vi "process.vi"(11 "class":refnum<class "selection_dropdown.lvclass">) -> ()   [LabVIEW 2024, in "selection_dropdown.lvclass"]
uses:
  selection_dropdown.lvclass
  refs.ctl
  selection_dropdown.lvclass/selection_dropdown.ctl
  <vilib>/addons/_JKI Toolkits/State Machine/_JKI_lib_State_Machine.llb/Select State(s)_err__jki_lib_state_machine.vi
  6cc69b80-9b04-4322-8415-f8fc40951971.vi
  <vilib>/addons/_JKI Toolkits/State Machine/_JKI_lib_State_Machine.llb/Periodic Trigger__ogtk__JKI-SM__jki_lib_state_machine.vi
  <vilib>/ErrorRing/Error Ring.xnode
panel:
  in  "Exit":bool
  in  "error in (no error)":errorcluster
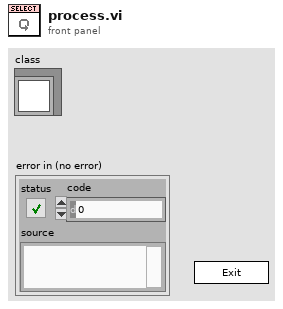
[diagram p1: front panel]
types:
  T1 = enum32{"Invalid", "Standard", "Closed", "Hidden", "Minimized", "Maximized"}
  T2 = enum32{"invalid app kind", "Development System", "Run Time System", "Student Edition", "Embedded LabVIEW", "Evaluation", "Custom"}
  T3 = typedef "selection_dropdown.lvclass/refs.ctl" = cluster{"selection":refnum<vi>, "cancel":refnum<vi>, "list":refnum<vi>, "available":refnum<vi>, "delete":refnum<vi>, "delete all":refnum<vi>}
  T4 = cluster{"Core":cluster{"Current VI Reference":refnum<vi>, "Close Panel on Exit?":bool}, "class":refnum<class "selection_dropdown.lvclass">, "refs":T3, "avail set":string[]}
  T5 = cluster{"Current VI Reference":refnum<vi>, "Close Panel on Exit?":bool}
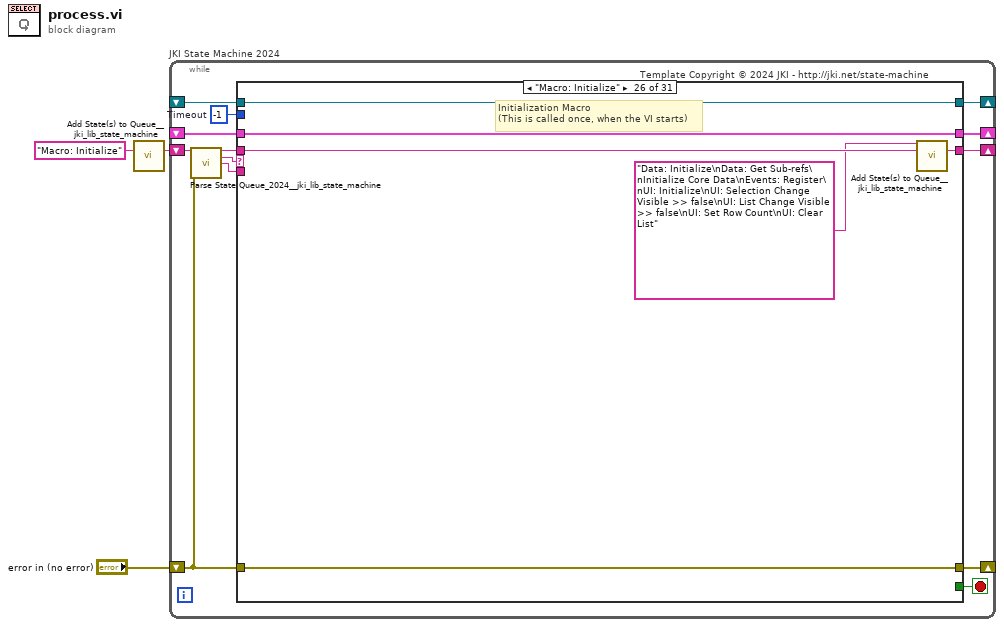
[diagram p0: block diagram]
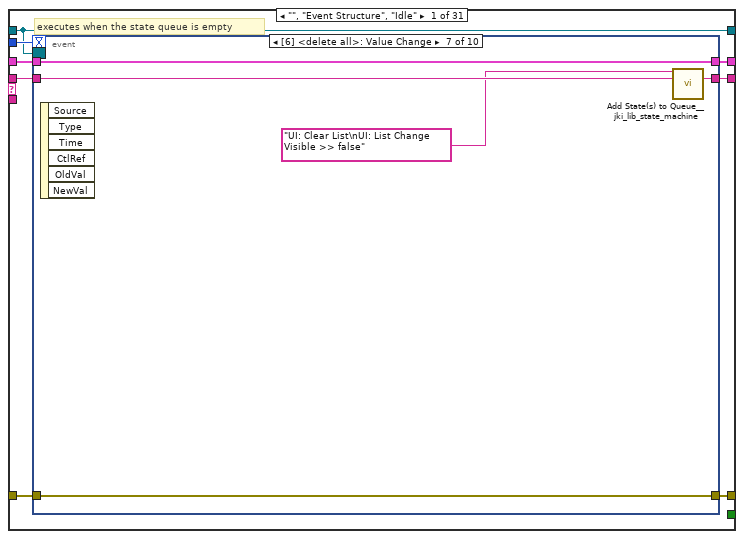
[diagram p2: hidden frame]
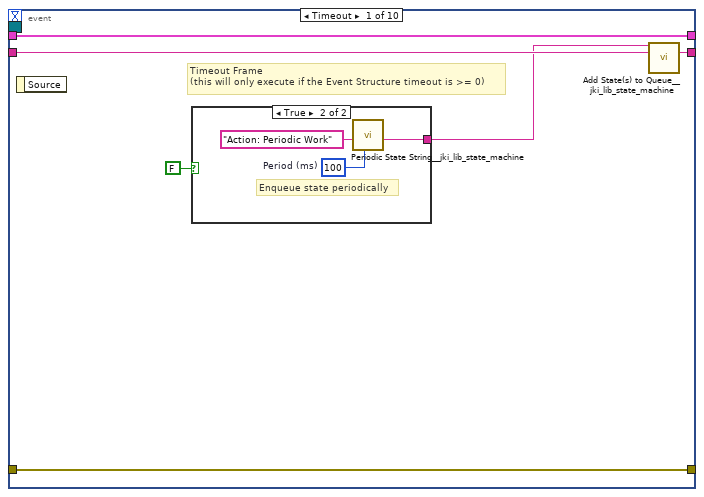
[diagram p3: hidden frame]
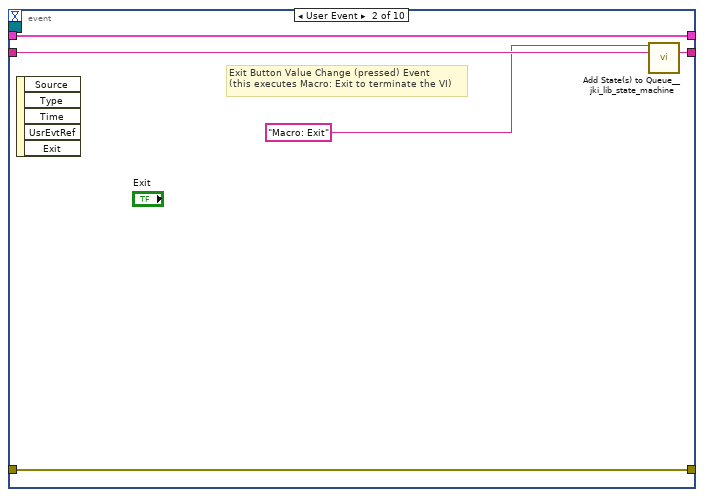
[diagram p5: hidden frame]
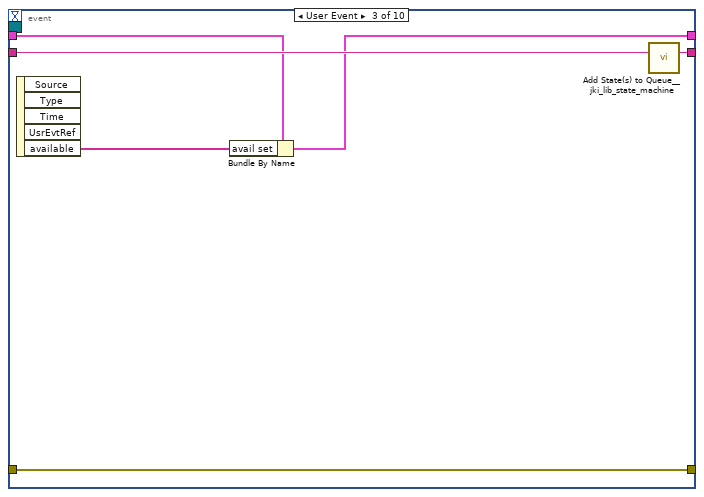
[diagram p6: hidden frame]
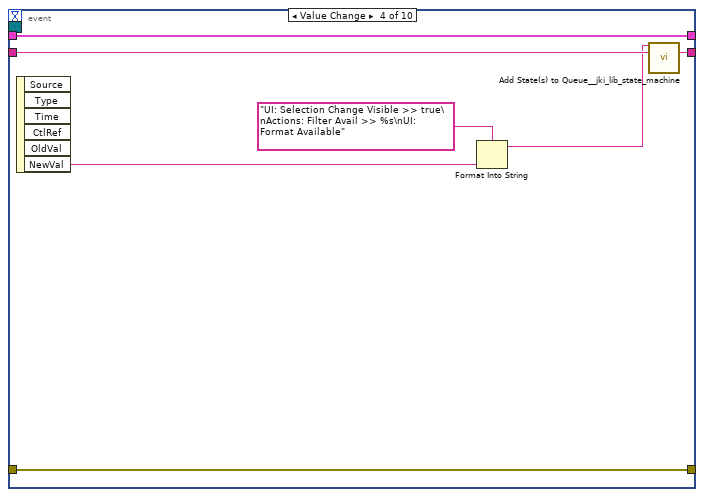
[diagram p7: hidden frame]
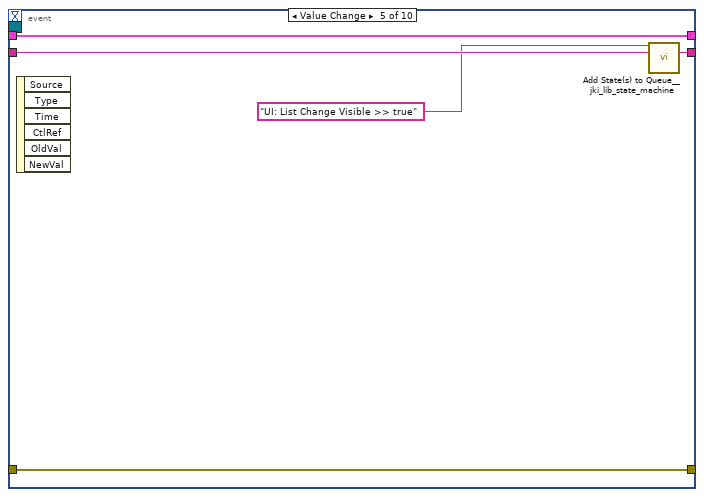
[diagram p8: hidden frame]
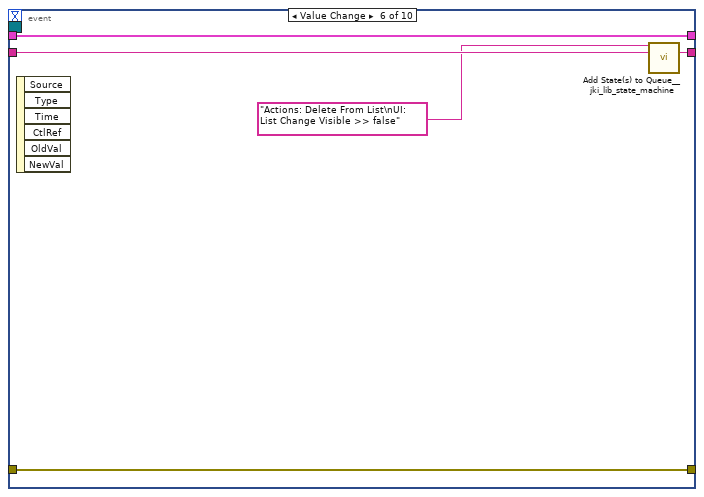
[diagram p9: hidden frame]
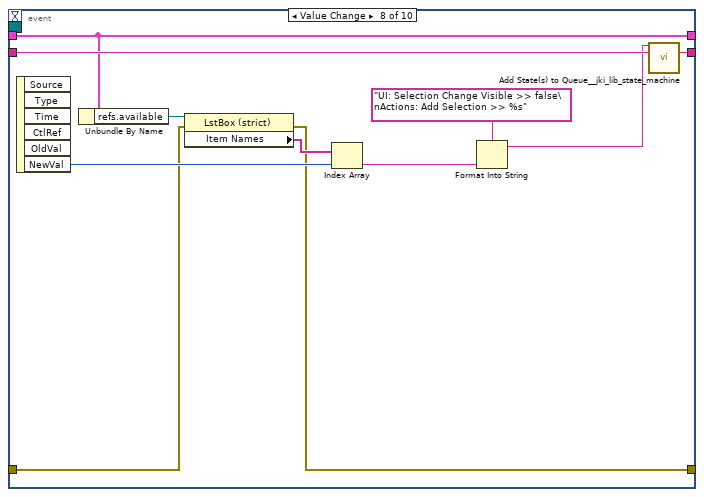
[diagram p10: hidden frame]
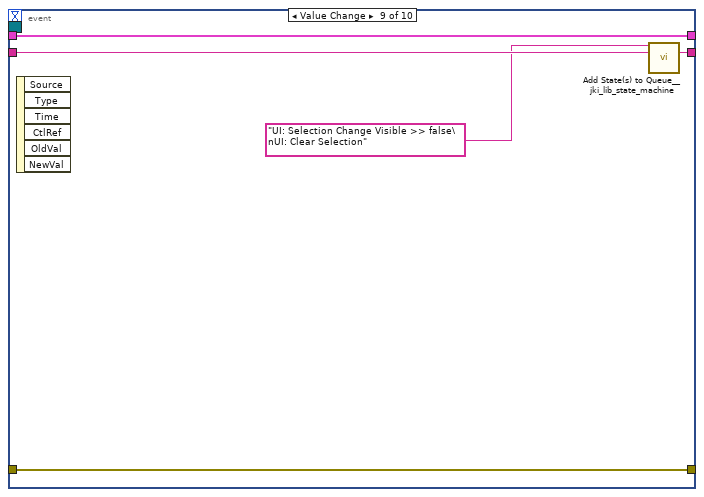
[diagram p11: hidden frame]
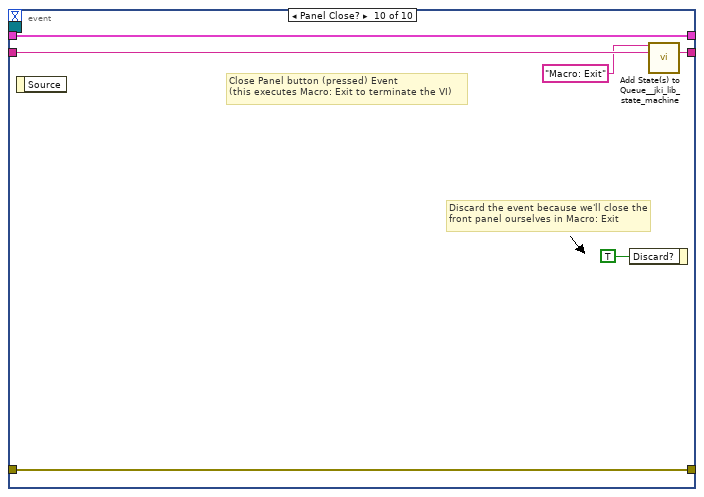
[diagram p12: hidden frame]
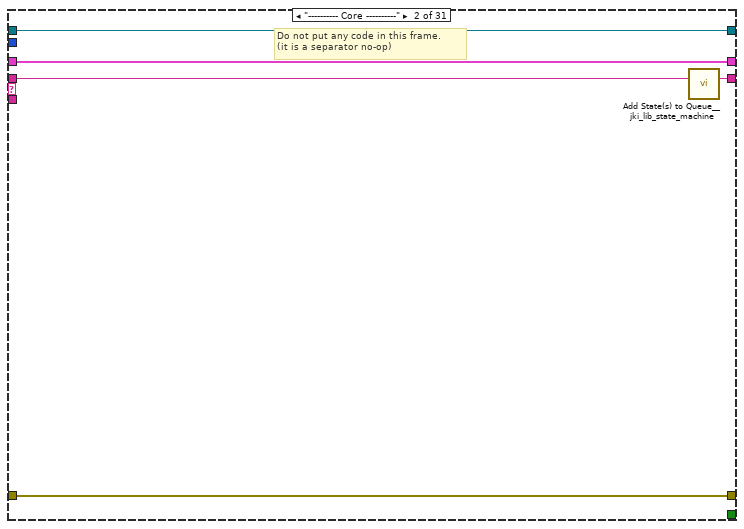
[diagram p13: hidden frame]
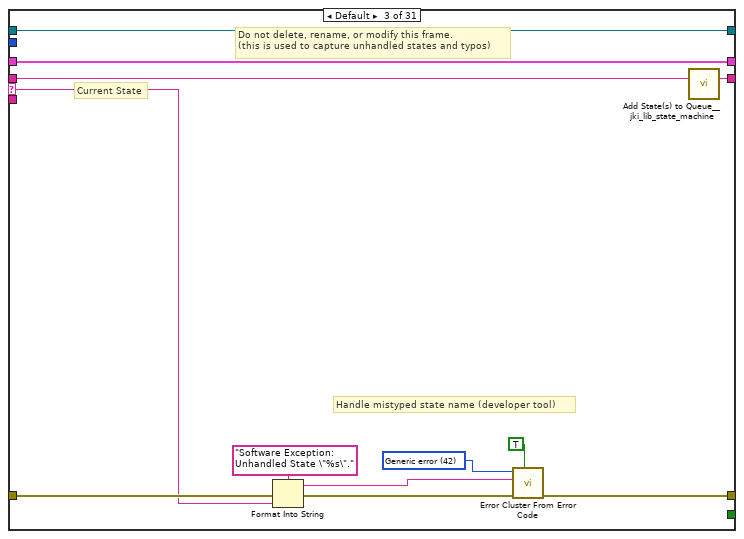
[diagram p14: hidden frame]
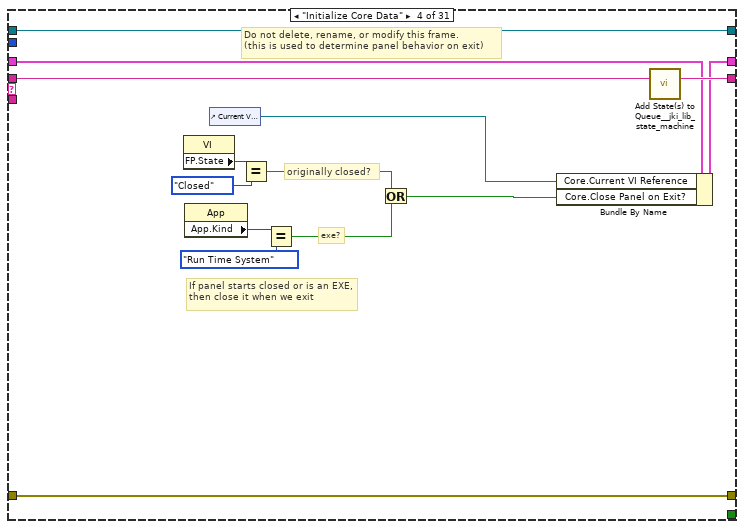
[diagram p15: hidden frame]
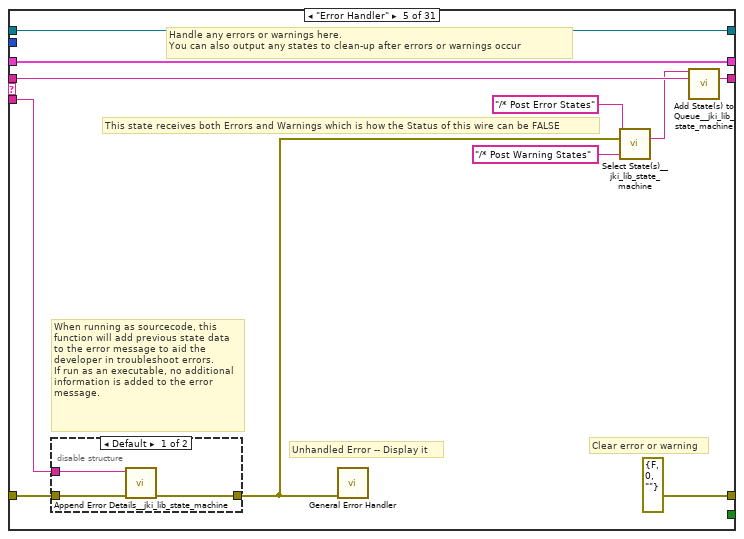
[diagram p16: hidden frame]
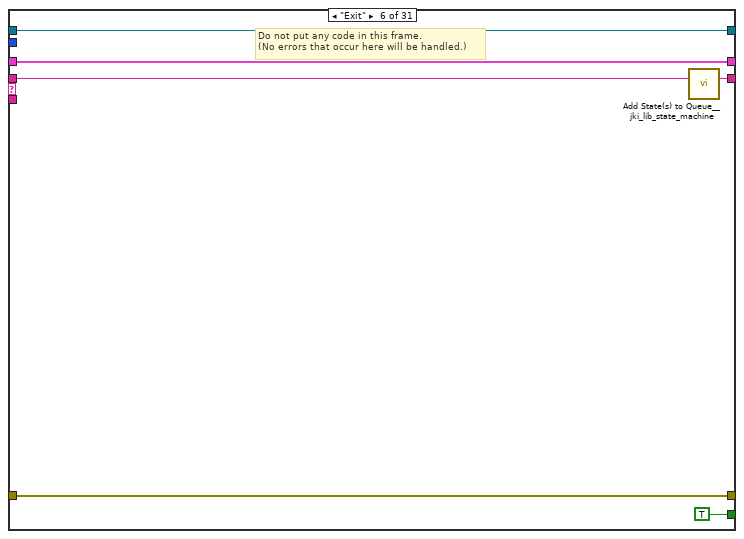
[diagram p18: hidden frame]
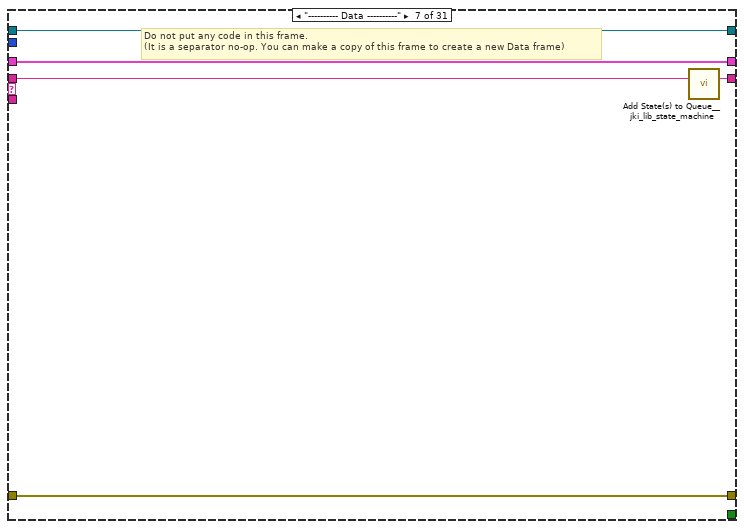
[diagram p19: hidden frame]
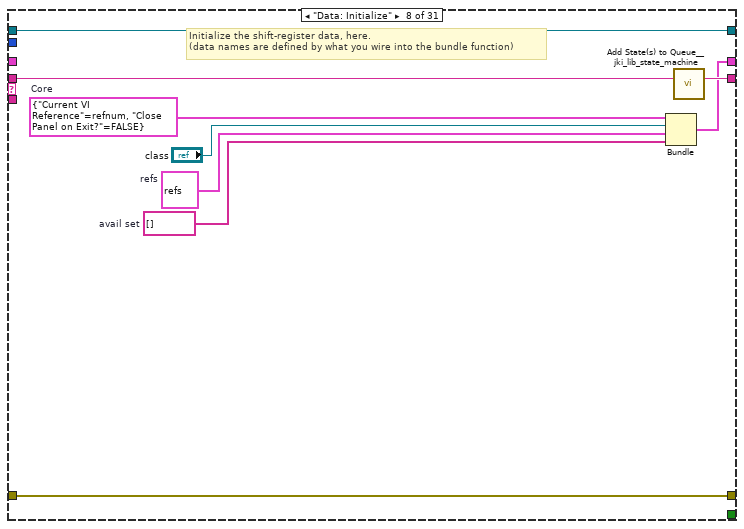
[diagram p20: hidden frame]
diagram:
  n1 = call <vilib>:"Add State(s) to Queue__jki_lib_state_machine.vi"("State(s) in (\"\")"="Macro: Initialize") -> ("States Out"=w3:string)  [unwired: 14 in]
  n2 = while "JKI State Machine 2024" {
    shift-right: [w9] -> _
    shift-left: _ -> [w8]
    shift-right: [w12] -> _
    shift-left: "error in (no error)" -> [w6]
    shift-right: [w11] -> _
    shift-left: w3 -> [w13]
    shift-right: [w5] -> _
    shift-left: _ -> [w4]
    stop <- w10 stop-if-true
    w7 = -1  # Timeout
    # "Template Copyright © 2024 JKI - http://jki.net/state-machine"
    n3 = call <vilib>:"Parse State Queue_2024__jki_lib_state_machine.vi"("State Queue"=w13, "Error In (no error)"=w6) -> ("Remaining States"=w15:string, "Current State"=w16:string, "Arguments"=w14:string)  [unwired: 11 in]
    n4 = case shown="\"Macro: Initialize\"" w16 {
      selector: w16 -> [_ _ w95 _ _ _ _ _ _ _ _ _ _ _ _ _ _ _ _ _ _ _ _ _ _ _ _ _ _ _ _]
      tunnel: w15 -> [w24 w93 w99 w119 w130 w140 w145 w154 w161 w179 w250 w265 w274 w279 w287 w292 w299 w311 w388 w400 w408 w420 w429 w448 w458 w464 w474 w479 w498 w514 w526]
      tunnel: w14 -> [_ _ _ _ w125 _ _ _ _ _ _ _ _ _ _ _ w294 w305 w383 w395 _ _ _ _ _ _ _ _ w492 _ w522]
      tunnel: w8 -> [w22 w90 w97 w112 w127 w138 w142 _ w156 w171 w247 w261 w271 w276 w284 w290 w297 w307 w386 w398 w406 w418 w427 w446 w455 w461 w472 w476 w495 w511 w523]
      tunnel: [w21 w91 w101 w116 errorcluster {"status"=FALSE, "code"=0, "source"=""} ("error out") w137 w143 w151 w157 w164 w248 w262 w266 w277 w280 w289 w295 w308 w377 w391 w402 w412 w423 w434 w456 w462 w469 w477 w483 w502 w519] -> w12
      tunnel: w6 -> [w18 w91 w100 w116 w126 w137 w143 w151 w158 w173 w248 w263 w268 w277 w281 w289 w296 w309 w379 w393 w403 w415 w424 w444 w456 w462 w469 w477 w488 w506 w520]
      tunnel: [w23 w92 w98 w118 w129 w139 w144 w153 w160 w178 w249 w264 w273 w278 w286 w291 w298 w310 w387 w399 w407 w419 w428 w447 w457 w463 w473 w478 w497 w513 w525] -> w11
      tunnel: [_ _ _ _ _ TRUE _ _ _ _ _ _ _ _ _ _ _ _ _ _ _ _ _ _ _ _ _ _ _ _ _] -> w10
      tunnel: [w20 w90 w97 w117 w127 w138 w142 w152 w156 w169 w247 w261 w271 w276 w284 w290 w297 w307 w386 w398 w406 w418 w427 w446 w455 w461 w472 w476 w495 w511 w523] -> w9
      tunnel: w7 -> [w19 _ _ _ _ _ _ _ _ _ _ _ _ _ _ _ _ _ _ _ _ _ _ _ _ _ _ _ _ _ _]
      tunnel: [w17 w89 w94 w106 w120 w135 w141 w149 w155 w177 w246 w252 w272 w275 w285 w288 w293 w304 w385 w397 w405 w417 w426 w445 w454 w459 w465 w475 w496 w512 w524] -> w5
      tunnel: w4 -> [w17 w89 w94 w106 w120 w135 w141 w149 w155 w177 w246 _ w272 w275 w285 w288 w293 w304 w385 w397 w405 w417 w426 w445 w454 w459 w465 w475 w496 w512 w524]
      frame "", "Event Structure", "Idle" {
        # "executes when the state queue is empty"
        n5 = event shown="[6] <delete all>: Value Change" {
          selector: w17 -> [_ _ _ _ _ _ _ _ _ _]
          dyn-events: _ -> [_ _ _ _ _ _ _ _ _ _]
          timeout: w19 -> [_ _ _ _ _ _ _ _ _ _]
          tunnel: w24 -> [w30 w38 w44 w51 w56 w61 w66 w77 w82 w88]
          tunnel: [w29 w37 w43 w50 w55 w60 w65 w76 w81 w87] -> w23
          tunnel: w22 -> [w27 w35 w41 w48 w53 w58 w63 w73 w79 w85]
          tunnel: [w28 w36 w42 w49 w54 w59 w64 w68 w80 w86] -> w21
          tunnel: w18 -> [w28 w36 w42 w49 w54 w59 w64 w67 w80 w86]
          tunnel: [w27 w35 w40 w48 w53 w58 w63 w73 w79 w85] -> w20
          event Timeout {
            # "Timeout Frame\n(this will only execute if the Event Structure timeout is >= 0)"
            n6 = event-data() -> ()  [unwired: 1 in, 1 out]
            n7 = case shown="True" FALSE {
              tunnel: [_ w33] -> w26
              frame False {
              }
              frame True {
                w31 = u32 100  # Period (ms)
                # "Enqueue state periodically"
                n8 = call <vilib>:"Periodic State String__jki_lib_state_machine.vi"("Period (ms)"=w31, "State"="Action: Periodic Work") -> ("State Out"=w33:string)  [unwired: 9 in]
              }
            }
            n9 = call <vilib>:"Add State(s) to Queue__jki_lib_state_machine.vi"("State(s) in Front (\"\")"=w26, "State(s) in (\"\")"=w30) -> ("States Out"=w29:string)  [unwired: 13 in]
          }
          event User Event {
            # "Exit Button Value Change (pressed) Event\n(this executes Macro: Exit to terminate the VI)"
            n10 = event-data() -> ()  [unwired: 1 in, 5 out]
            n11 = call <vilib>:"Add State(s) to Queue__jki_lib_state_machine.vi"("State(s) in Front (\"\")"="Macro: Exit", "State(s) in (\"\")"=w38) -> ("States Out"=w37:string)  [unwired: 13 in]
          }
          event User Event {
            n12 = event-data() -> ("available"=w39:string[])  [unwired: 1 in, 4 out]
            n13 = Bundle By Name(cluster=w41, "avail set"=w39) -> (w40:T4)
            n14 = call <vilib>:"Add State(s) to Queue__jki_lib_state_machine.vi"("State(s) in (\"\")"=w44) -> ("States Out"=w43:string)  [unwired: 14 in]
          }
          event Value Change {
            n15 = event-data() -> ("NewVal"=w46:string)  [unwired: 1 in, 5 out]
            n16 = Format Into String(format string="UI: Selection Change Visible >> true\nActions: Filter Avail >> %s\nUI: Format Available", w46) -> (resulting string=w45:string)  [unwired: 2 in, 1 out]
            n17 = call <vilib>:"Add State(s) to Queue__jki_lib_state_machine.vi"("State(s) in Front (\"\")"=w45, "State(s) in (\"\")"=w51) -> ("States Out"=w50:string)  [unwired: 13 in]
          }
          event Value Change {
            n18 = event-data() -> ()  [unwired: 1 in, 6 out]
            n19 = call <vilib>:"Add State(s) to Queue__jki_lib_state_machine.vi"("State(s) in Front (\"\")"="UI: List Change Visible >> true", "State(s) in (\"\")"=w56) -> ("States Out"=w55:string)  [unwired: 13 in]
          }
          event Value Change {
            n20 = event-data() -> ()  [unwired: 1 in, 6 out]
            n21 = call <vilib>:"Add State(s) to Queue__jki_lib_state_machine.vi"("State(s) in Front (\"\")"="Actions: Delete From List\nUI: List Change Visible >> false", "State(s) in (\"\")"=w61) -> ("States Out"=w60:string)  [unwired: 13 in]
          }
          event Value Change {
            n22 = event-data() -> ()  [unwired: 1 in, 6 out]
            n23 = call <vilib>:"Add State(s) to Queue__jki_lib_state_machine.vi"("State(s) in Front (\"\")"="UI: Clear List\nUI: List Change Visible >> false", "State(s) in (\"\")"=w66) -> ("States Out"=w65:string)  [unwired: 13 in]
          }
          event Value Change {
            n24 = event-data() -> ("NewVal"=w72:i32)  [unwired: 1 in, 5 out]
            n25 = Unbundle By Name(w73) -> ("refs.available"=w70:refnum<vi>)
            n26 = property class="LstBox (strict)"(reference=w70, error in=w67) -> (error out=w68:errorcluster, "Item Names"=w69:string[])  [unwired: 1 out]
            n27 = Index Array(array=w69, index=w72) -> (element=w71:string)
            n28 = Format Into String(format string="UI: Selection Change Visible >> false\nActions: Add Selection >> %s", w71) -> (resulting string=w74:string)  [unwired: 2 in, 1 out]
            n29 = call <vilib>:"Add State(s) to Queue__jki_lib_state_machine.vi"("State(s) in Front (\"\")"=w74, "State(s) in (\"\")"=w77) -> ("States Out"=w76:string)  [unwired: 13 in]
          }
          event Value Change {
            n30 = event-data() -> ()  [unwired: 1 in, 6 out]
            n31 = call <vilib>:"Add State(s) to Queue__jki_lib_state_machine.vi"("State(s) in Front (\"\")"="UI: Selection Change Visible >> false\nUI: Clear Selection", "State(s) in (\"\")"=w82) -> ("States Out"=w81:string)  [unwired: 13 in]
          }
          event Panel Close? {
            # "Discard the event because we'll close the front panel ourselves in Macro: Exit"
            # "Close Panel button (pressed) Event\n(this executes Macro: Exit to terminate the VI)"
            n32 = event-data() -> ()  [unwired: 1 in, 1 out]
            n33 = event-data("Discard?"=TRUE) -> ()  [unwired: 1 in, 1 out]
            n34 = call <vilib>:"Add State(s) to Queue__jki_lib_state_machine.vi"("State(s) in Front (\"\")"="Macro: Exit", "State(s) in (\"\")"=w88) -> ("States Out"=w87:string)  [unwired: 13 in]
          }
        }
      }
      frame "---------- Core ----------" {
        # "Do not put any code in this frame.\n(it is a separator no-op)"
        n35 = call <vilib>:"Add State(s) to Queue__jki_lib_state_machine.vi"("State(s) in (\"\")"=w93) -> ("States Out"=w92:string)  [unwired: 14 in]
      }
      frame Default {
        w104 = 42 items=["No error", "Argument error", "Memory is full", "Out of zone", "End of file", "File already open", "Generic file I/O error", "File not found", "File permission error", "Disk is full", "Duplicate path", "Too many files open", "System feature not enabled", "Resource file not found", "Cannot add resource", "Resource not found", "Image not found", "Image memory error", "Pen does not exist", "Config type invalid", "Config token not found", "Config parse error", "Config memory error", "Bad external code format", "Bad external code offset", "External code not present", "Null window", "Destroy window error", "Null menu", "Print aborted", "Bad print record", "Print driver error", "Windows error during printing", "Memory error during printing", "Print dialog error", "Generic print error", "Invalid device refnum", "Device not found", "Device parameter error", "Device unit error", "Cannot open device", "Device call aborted", "Generic error", "Cancelled by user", "Object ID too low", "Object ID too high", "Object not in heap", "Unknown heap", "Unknown object (invalid DefProc)", "Unknown object (DefProc not in table)", "Message out of range", "Invalid (null) method", "Unknown message", "Manager call not supported", "Bad address", "Network operation in progress", "Network operation timed out", "Connection is busy", "Network attribute not supported", "Network error", "Address in use", "System out of memory", "Connection aborted", "Connection refused", "Not connected", "Already connected", "Connection closed", "Initialization error (interapplication manager)", "Bad occurrence", "Wait on unbound occurrence handler", "Occurrence queue overflow", "Datalog type conflict", "Unused", "Unrecognized type (interapplication manager)", "Memory corrupt", "Failed to make temporary DLL", "Old CIN version", "Drag socket not found", "Failed to load drop-object", "Failed to register OLE object", "Failed to release OLE object", "Format specifier type mismatch", "Unknown format specifier", "Too few format specifiers", "Too many format specifiers", "Scan failed", "Newer CIN version", "Error converting to variant", "Runtime menu error", "Password tampered", "Variant attribute not found", "Incompatible variant data type", "Event data is not available", "Event Store is not present", "Occurrence is not found", "Event Queue is not created", "Event info is not available", "Refnum passed is NULL", "Error retrieving Class GUID", "Error retrieving CoClass GUID", "Error retrieving TypeLib GUID.", "Bad built application magic bytes.", "Specific driver is different from the specific driver associated with the Logical Name.", "There is no session opened to the class driver.", "Max Error", "MAX - Error with config objects", "MAX - Error loading configuration", "MAX - Group not supported"]
        # "Current State"
        # "Do not delete, rename, or modify this frame.\n(this is used to capture unhandled states and typos)"
        # "Handle mistyped state name (developer tool)"
        n36 = Format Into String(format string="Software Exception: Unhandled State \"%s\"." ("message"), error in=w100, w95) -> (resulting string=w103:string, error out=w102:errorcluster)  [unwired: 1 in]
        n37 = call <vilib>:"Error Cluster From Error Code.vi"("show call chain? (False)"=TRUE, "error in (no error)"=w102, "error message (\"\")"=w103, "error code (0)"=w104) -> ("error out"=w101:errorcluster)  [unwired: 5 in]
        n38 = call <vilib>:"Add State(s) to Queue__jki_lib_state_machine.vi"("State(s) in (\"\")"=w99) -> ("States Out"=w98:string)  [unwired: 14 in]
      }
      frame "Initialize Core Data" {
        # "Do not delete, rename, or modify this frame.\n(this is used to determine panel behavior on exit)"
        # "originally closed?"
        # "exe?"
        # "If panel starts closed or is an EXE, then close it when we exit"
        n39 = property class="VI"() -> ("FP.State"=w109:T1)  [unwired: 2 in, 2 out]
        n40 = property class="App"() -> ("App.Kind"=w115:T2)  [unwired: 2 in, 2 out]
        n41 = control-ref of="Current VI Reference"() -> (w110:refnum<vi>)
        n42 = Equal?(x=w109, y=T1."Closed" ("Front Panel Window:State")) -> (x = y?=w107:bool)
        n43 = Equal?(x=w115, y=T2."Run Time System" ("Application:Kind")) -> (x = y?=w113:bool)
        n44 = Or(x=w107, y=w113) -> (x .or. y?=w111:bool)
        n45 = Bundle By Name(cluster=w112, "Core.Current VI Reference"=w110, "Core.Close Panel on Exit?"=w111) -> (w117:T4)
        n46 = call <vilib>:"Add State(s) to Queue__jki_lib_state_machine.vi"("State(s) in (\"\")"=w119) -> ("States Out"=w118:string)  [unwired: 14 in]
      }
      frame "Error Handler" {
        # "When running as sourcecode, this function will add previous state data to the error message to aid the developer in troubleshoot errors.\nIf run as an executable, no additional information is added to the error message."
        # "This state receives both Errors and Warnings which is how the Status of this wire can be FALSE"
        # "Unhandled Error -- Display it"
        # "Handle any errors or warnings here.\nYou can also output any states to clean-up after errors or warnings occur"
        # "Clear error or warning"
        n47 = disable-structure shown="Default" {
          disable-tunnel: w126 -> [w133 w134]
          disable-tunnel: w125 -> [w132 _]
          disable-tunnel: [w131 w134] -> w124
          frame condition #0 (active) {
            n48 = call <vilib>:"Append Error Details__jki_lib_state_machine.vi"("error in (no error)"=w133, "Previous State and Argument(s)"=w132) -> ("error out"=w131:errorcluster)  [unwired: 9 in]
          }
          frame condition #1 {
          }
        }
        n49 = call <vilib>:"General Error Handler.vi"("error in (no error)"=w124) -> ()  [unwired: 10 in, 5 out]
        n50 = call-poly <vilib>:"Select State(s)__jki_lib_state_machine.vi"("State(s) if True (\"\")"="/* Post Error States", "Select"=w124, "State(s) if False (\"\")"="/* Post Warning States") -> ("States Out"=w122:string)  [unwired: 12 in]
        n51 = call <vilib>:"Add State(s) to Queue__jki_lib_state_machine.vi"("State(s) in Front (\"\")"=w122, "State(s) in (\"\")"=w130) -> ("States Out"=w129:string)  [unwired: 13 in]
      }
      frame "Exit" {
        # "Do not put any code in this frame.\n(No errors that occur here will be handled.)"
        n52 = call <vilib>:"Add State(s) to Queue__jki_lib_state_machine.vi"("State(s) in (\"\")"=w140) -> ("States Out"=w139:string)  [unwired: 14 in]
      }
      frame "---------- Data ----------" {
        # "Do not put any code in this frame.\n(It is a separator no-op. You can make a copy of this frame to create a new Data frame)"
        n53 = call <vilib>:"Add State(s) to Queue__jki_lib_state_machine.vi"("State(s) in (\"\")"=w145) -> ("States Out"=w144:string)  [unwired: 14 in]
      }
      frame "Data: Initialize" {
        w146 = string[] []  # avail set
        w147 = T3 {"selection"=refnum, "cancel"=refnum, "list"=refnum, "available"=refnum, "delete"=refnum, "delete all"=refnum}  # refs
        w150 = T5 {"Current VI Reference"=refnum, "Close Panel on Exit?"=FALSE}  # Core
        # "Initialize the shift-register data, here.\n(data names are defined by what you wire into the bundle function)"
        n54 = Bundle("Core"=w150, "class"="class", "refs"=w147, "avail set"=w146) -> (w152:T4)  [unwired: 1 in]
        n55 = call <vilib>:"Add State(s) to Queue__jki_lib_state_machine.vi"("State(s) in (\"\")"=w154) -> ("States Out"=w153:string)  [unwired: 14 in]
      }
      frame "Data: Cleanup" {
        # "Cleanup any data and references, here.\n(this is called automatically, by the Macro: Exit)"
        n56 = Unbundle By Name(w156) -> ("Core.Current VI Reference"=w159:refnum<vi>)
        n57 = Close Reference(reference=w159, error in (no error)=w158) -> (error out=w157:errorcluster)
        n58 = call <vilib>:"Add State(s) to Queue__jki_lib_state_machine.vi"("State(s) in (\"\")"=w161) -> ("States Out"=w160:string)  [unwired: 14 in]
      }
      frame "Data: Get Sub-refs" {
        n59 = Unbundle By Name(w171) -> ("class"=w176:refnum<class "selection_dropdown.lvclass">)
        n60 = Unbundle By Name(w171) -> ("refs.delete all"=w162:refnum<vi>, "refs.selection"=w170:refnum<vi>, "refs.cancel"=w168:refnum<vi>, "refs.list"=w167:refnum<vi>, "refs.available"=w166:refnum<vi>, "refs.delete"=w165:refnum<vi>)
        n61 = Unbundle By Name(w176) -> ("ref"=w175:refnum<vi>)
        n62 = property class="Clust (strict)"(reference=w175, error in=w173) -> (error out=w172:errorcluster, "Controls[]"=w174:refnum<vi>[])  [unwired: 1 out]
        n63 = xnode "Error Ring"() -> ("error out"=w163:errorcluster)
        n64 = for {
          tunnel: w174 -> [w199] mode=indexing
          shift-right: [w192] -> w164
          shift-left: w172 -> [w197]
          tunnel: w170 -> [w193]
          shift-right: [w191] -> w169
          shift-left: w171 -> [w194]
          tunnel: w168 -> [w190]
          tunnel: w167 -> [w189]
          tunnel: w166 -> [w188]
          tunnel: w165 -> [w187]
          tunnel: w163 -> [w186]
          tunnel: w162 -> [w185]
          n65 = property class="Ctl"(reference=w199, error in=w197) -> (reference out=w195:refnum<vi>, error out=w196:errorcluster, "Label.Text"=w198:string)
          n66 = case shown="\"delete all\"" w198 {
            tunnel: w196 -> [w206 w213 w220 w227 w234 w241 w242]
            tunnel: w195 -> [w205 w212 w219 w226 w233 w240 _]
            tunnel: w194 -> [w203 w211 w218 w225 w232 w239 w245]
            tunnel: w193 -> [w204 _ _ _ _ _ _]
            tunnel: [w201 w209 w216 w223 w230 w237 w244] -> w192
            tunnel: [w200 w208 w215 w222 w229 w236 w245] -> w191
            tunnel: w190 -> [_ w207 _ _ _ _ _]
            tunnel: w189 -> [_ _ w214 _ _ _ _]
            tunnel: w188 -> [_ _ _ w221 _ _ _]
            tunnel: w187 -> [_ _ _ _ w228 _ _]
            tunnel: w186 -> [_ _ _ _ _ _ w243]
            tunnel: w185 -> [_ _ _ _ _ w235 _]
            frame "selection" {
              n67 = To More Specific Class(target class=w204, reference=w205, error in=w206) -> (specific class reference=w202:refnum<vi>, error out=w201:errorcluster)
              n68 = Bundle By Name(cluster=w203, "refs.selection"=w202) -> (w200:T4)
            }
            frame "cancel" {
              n69 = To More Specific Class(target class=w207, reference=w212, error in=w213) -> (specific class reference=w210:refnum<vi>, error out=w209:errorcluster)
              n70 = Bundle By Name(cluster=w211, "refs.cancel"=w210) -> (w208:T4)
            }
            frame "list" {
              n71 = To More Specific Class(target class=w214, reference=w219, error in=w220) -> (specific class reference=w217:refnum<vi>, error out=w216:errorcluster)
              n72 = Bundle By Name(cluster=w218, "refs.list"=w217) -> (w215:T4)
            }
            frame "available" {
              n73 = To More Specific Class(target class=w221, reference=w226, error in=w227) -> (specific class reference=w224:refnum<vi>, error out=w223:errorcluster)
              n74 = Bundle By Name(cluster=w225, "refs.available"=w224) -> (w222:T4)
            }
            frame "delete" {
              n75 = To More Specific Class(target class=w228, reference=w233, error in=w234) -> (specific class reference=w231:refnum<vi>, error out=w230:errorcluster)
              n76 = Bundle By Name(cluster=w232, "refs.delete"=w231) -> (w229:T4)
            }
            frame "delete all" {
              n77 = To More Specific Class(target class=w235, reference=w240, error in=w241) -> (specific class reference=w238:refnum<vi>, error out=w237:errorcluster)
              n78 = Bundle By Name(cluster=w239, "refs.delete all"=w238) -> (w236:T4)
            }
            frame Default {
              n79 = Merge Errors(w242, w243) -> (w244:errorcluster)
            }
          }
        }
        n80 = call <vilib>:"Add State(s) to Queue__jki_lib_state_machine.vi"("State(s) in (\"\")"=w179) -> ("States Out"=w178:string)  [unwired: 14 in]
      }
      frame "---------- Events ----------" {
        # "Do not put any code in this frame.\n(It is a separator no-op. You can make a copy of this frame to create a new UI frame)"
        n81 = call <vilib>:"Add State(s) to Queue__jki_lib_state_machine.vi"("State(s) in (\"\")"=w250) -> ("States Out"=w249:string)  [unwired: 14 in]
      }
      frame "Events: Register" {
        n82 = Unbundle By Name(w261) -> ("class"=w260:refnum<class "selection_dropdown.lvclass">)
        n83 = Unbundle By Name(w260) -> ("avail set event"=w256:refnum<user-event>, "exit event"=w259:refnum<user-event>)
        n84 = Unbundle By Name(w261) -> ("refs.selection"=w258:refnum<vi>, "refs.cancel"=w257:refnum<vi>, "refs.available"=w255:refnum<vi>, "refs.list"=w254:refnum<vi>, "refs.delete"=w253:refnum<vi>, "refs.delete all"=w251:refnum<vi>)
        n85 = register-events(error in=w263, w256, w259, w258, w257, w255, w254, w253, w251) -> (reference out=w252:refnum<event-registration>, error out=w262:errorcluster)  [unwired: 1 in]
        n86 = call <vilib>:"Add State(s) to Queue__jki_lib_state_machine.vi"("State(s) in (\"\")"=w265) -> ("States Out"=w264:string)  [unwired: 14 in]
      }
      frame "Events: Unregister" {
        n87 = Unregister For Events(event registration refnum=w272, error in=w268) -> (error out=w267:errorcluster)
        n88 = Unbundle By Name(w271) -> ("class"=w270:refnum<class "selection_dropdown.lvclass">)
        n89 = Unbundle By Name(w270) -> ("exit event"=w269:refnum<user-event>)
        n90 = Destroy User Event(user event=w269, error in=w267) -> (error out=w266:errorcluster)
        n91 = call <vilib>:"Add State(s) to Queue__jki_lib_state_machine.vi"("State(s) in (\"\")"=w274) -> ("States Out"=w273:string)  [unwired: 14 in]
      }
      frame "---------- UI ----------" {
        # "Do not put any code in this frame.\n(It is a separator no-op. You can make a copy of this frame to create a new UI frame)"
        n92 = call <vilib>:"Add State(s) to Queue__jki_lib_state_machine.vi"("State(s) in (\"\")"=w279) -> ("States Out"=w278:string)  [unwired: 14 in]
      }
      frame "UI: Initialize" {
        n93 = Unbundle By Name(w284) -> ("refs.selection"=w283:refnum<vi>)
        n94 = property class="Str"(reference=w283, error in=w281, "Value"="") -> (error out=w280:errorcluster)  [unwired: 1 out]
        n95 = call <vilib>:"Add State(s) to Queue__jki_lib_state_machine.vi"("State(s) in (\"\")"=w287) -> ("States Out"=w286:string)  [unwired: 14 in]
      }
      frame "UI: Uninitialize" {
        # "Cleanup the User Interface, here.\n(this is called automatically, by the Macro: Exit)"
        n96 = call <vilib>:"Add State(s) to Queue__jki_lib_state_machine.vi"("State(s) in (\"\")"=w292) -> ("States Out"=w291:string)  [unwired: 14 in]
      }
      frame "UI: Cursor Set" {
        # "Argument"
        # "Set and Unset Cursor Busy.\n(Usage: \"UI: Cursor Set >> Busy|Idle\")"
        n97 = case shown="\"Idle\", Default" w294 {
          tunnel: w296 -> [w301 w303]
          tunnel: [w300 w302] -> w295
          frame "Idle", Default {
            n98 = call <vilib>:"Unset Busy.vi"("error in (no error)"=w301) -> ("error out"=w300:errorcluster)  [unwired: 10 in]
          }
          frame "Busy" {
            n99 = call <vilib>:"Set Busy.vi"("error in (no error)"=w303) -> ("error out"=w302:errorcluster)  [unwired: 9 in, 1 out]
          }
        }
        n100 = call <vilib>:"Add State(s) to Queue__jki_lib_state_machine.vi"("State(s) in (\"\")"=w299) -> ("States Out"=w298:string)  [unwired: 14 in]
      }
      frame "UI: Front Panel State" {
        # "Argument"
        # "Set Front Panel Open or Closed\n(Usage: \"UI: Front Panel State >> Open|Close\")"
        n101 = Unbundle By Name(w307) -> ("Core.Current VI Reference"=w306:refnum<vi>)
        n102 = case shown="\"Open\", \"Standard\", Default" w305 {
          tunnel: w309 -> [w317 w332 w343 w356 w369]
          tunnel: [w319 w333 w345 w358 w371] -> w308
          tunnel: w306 -> [w318 w330 w344 w357 w370]
          frame "Open", "Standard", Default {
            w312 = T1."Standard" ("State")
            n103 = property class="VI"(reference=w318, error in=w317) -> (reference out=w315:refnum<vi>, error out=w316:errorcluster, "FP.State"=w314:T1)
            n104 = Not Equal?(x=w314, y=w312) -> (x != y?=w313:bool)
            n105 = case shown="True" w313 {
              tunnel: [w323 w325] -> w319
              tunnel: w316 -> [w322 w325]
              tunnel: w315 -> [w321 _]
              tunnel: w312 -> [w320 _]
              frame True {
                n106 = invoke class="VI" method="FP.Open"(reference=w321, error in=w322, "Activate"=TRUE, "State"=w320) -> (error out=w323:errorcluster)  [unwired: 1 in, 4 out]
              }
              frame False {
              }
            }
          }
          frame "Close", "Closed" {
            n107 = property class="VI"(reference=w330, error in=w332) -> (reference out=w329:refnum<vi>, error out=w331:errorcluster, "FP.State"=w327:T1)
            n108 = Not Equal?(x=w327, y=T1."Closed" ("Front Panel Window:State")) -> (x != y?=w326:bool)
            n109 = case shown="True" w326 {
              tunnel: [w334 w337] -> w333
              tunnel: w331 -> [w334 w336]
              tunnel: w329 -> [_ w335]
              frame False {
              }
              frame True {
                n110 = invoke class="VI" method="FP.Close"(reference=w335, error in=w336) -> (error out=w337:errorcluster)  [unwired: 1 in, 2 out]
              }
            }
          }
          frame "Hidden", "Hide" {
            w338 = T1."Hidden" ("State")
            n111 = property class="VI"(reference=w344, error in=w343) -> (reference out=w341:refnum<vi>, error out=w342:errorcluster, "FP.State"=w340:T1)
            n112 = Not Equal?(x=w340, y=w338) -> (x != y?=w339:bool)
            n113 = case shown="True" w339 {
              tunnel: [w349 w350] -> w345
              tunnel: w342 -> [w348 w350]
              tunnel: w341 -> [w347 _]
              tunnel: w338 -> [w346 _]
              frame True {
                n114 = invoke class="VI" method="FP.Open"(reference=w347, error in=w348, "State"=w346) -> (error out=w349:errorcluster)  [unwired: 2 in, 4 out]
              }
              frame False {
              }
            }
          }
          frame "Minimize", "Minimized" {
            w351 = T1."Minimized" ("State")
            n115 = property class="VI"(reference=w357, error in=w356) -> (reference out=w354:refnum<vi>, error out=w355:errorcluster, "FP.State"=w353:T1)
            n116 = Not Equal?(x=w353, y=w351) -> (x != y?=w352:bool)
            n117 = case shown="True" w352 {
              tunnel: [w362 w363] -> w358
              tunnel: w355 -> [w361 w363]
              tunnel: w354 -> [w360 _]
              tunnel: w351 -> [w359 _]
              frame True {
                n118 = invoke class="VI" method="FP.Open"(reference=w360, error in=w361, "State"=w359) -> (error out=w362:errorcluster)  [unwired: 2 in, 4 out]
              }
              frame False {
              }
            }
          }
          frame "Maximize", "Maximized" {
            w364 = T1."Maximized" ("State")
            n119 = property class="VI"(reference=w370, error in=w369) -> (reference out=w367:refnum<vi>, error out=w368:errorcluster, "FP.State"=w366:T1)
            n120 = Not Equal?(x=w366, y=w364) -> (x != y?=w365:bool)
            n121 = case shown="True" w365 {
              tunnel: [w375 w376] -> w371
              tunnel: w368 -> [w374 w376]
              tunnel: w367 -> [w373 _]
              tunnel: w364 -> [w372 _]
              frame True {
                n122 = invoke class="VI" method="FP.Open"(reference=w373, error in=w374, "State"=w372) -> (error out=w375:errorcluster)  [unwired: 2 in, 4 out]
              }
              frame False {
              }
            }
          }
        }
        n123 = call <vilib>:"Add State(s) to Queue__jki_lib_state_machine.vi"("State(s) in (\"\")"=w311) -> ("States Out"=w310:string)  [unwired: 14 in]
      }
      frame "UI: Selection Change Visible" {
        n124 = Unbundle By Name(w386) -> ("refs.cancel"=w381:refnum<vi>, "refs.available"=w382:refnum<vi>)
        n125 = Equal?(x=w383, y="true") -> (x = y?=w380:bool)
        n126 = property class="LstBox (strict)"(reference=w382, error in=w379, "Visible"=w380) -> (error out=w378:errorcluster)  [unwired: 1 out]
        n127 = property class="Bool (strict)"(reference=w381, error in=w378, "Visible"=w380) -> (error out=w377:errorcluster)  [unwired: 1 out]
        n128 = call <vilib>:"Add State(s) to Queue__jki_lib_state_machine.vi"("State(s) in (\"\")"=w388) -> ("States Out"=w387:string)  [unwired: 14 in]
      }
      frame "UI: List Change Visible" {
        n129 = Unbundle By Name(w398) -> ("refs.delete all"=w392:refnum<vi>, "refs.delete"=w394:refnum<vi>)
        n130 = Equal?(x=w395, y="true") -> (x = y?=w389:bool)
        n131 = property class="Bool (strict)"(reference=w394, error in=w393, "Visible"=w389) -> (error out=w390:errorcluster)  [unwired: 1 out]
        n132 = property class="Bool (strict)"(reference=w392, error in=w390, "Visible"=w389) -> (error out=w391:errorcluster)  [unwired: 1 out]
        n133 = call <vilib>:"Add State(s) to Queue__jki_lib_state_machine.vi"("State(s) in (\"\")"=w400) -> ("States Out"=w399:string)  [unwired: 14 in]
      }
      frame "UI: Clear Selection" {
        n134 = Unbundle By Name(w406) -> ("refs.selection"=w404:refnum<vi>)
        n135 = property class="Str"(reference=w404, error in=w403, "Value"="") -> (error out=w402:errorcluster)  [unwired: 1 out]
        n136 = call <vilib>:"Add State(s) to Queue__jki_lib_state_machine.vi"("State(s) in (\"\")"=w408) -> ("States Out"=w407:string)  [unwired: 14 in]
      }
      frame "UI: Clear List" {
        w409 = string[] [] ("Item Names")
        n137 = Unbundle By Name(w418) -> ("class"=w411:refnum<class "selection_dropdown.lvclass">, "refs.list"=w416:refnum<vi>)
        n138 = Unbundle By Name(w411) -> ("filter list event"=w410:refnum<user-event>)
        n139 = property class="LstBox (strict)"(reference=w416, error in=w415, "Value"=-1, "Item Names"=w409) -> (error out=w413:errorcluster)  [unwired: 1 out]
        n140 = Generate User Event(user event=w410, event data cluster=w409, error in=w413) -> (error out=w412:errorcluster)  [unwired: 1 in, 1 out]
        n141 = call <vilib>:"Add State(s) to Queue__jki_lib_state_machine.vi"("State(s) in (\"\")"=w420) -> ("States Out"=w419:string)  [unwired: 14 in]
      }
      frame "UI: Set Row Count" {
        n142 = Unbundle By Name(w427) -> ("refs.list"=w425:refnum<vi>, "class"=w422:refnum<class "selection_dropdown.lvclass">)
        n143 = Unbundle By Name(w422) -> ("Number of Rows"=w421:u32)
        n144 = property class="LstBox (strict)"(reference=w425, error in=w424, "Number of Rows"=w421) -> (error out=w423:errorcluster)  [unwired: 1 out]
        n145 = call <vilib>:"Add State(s) to Queue__jki_lib_state_machine.vi"("State(s) in (\"\")"=w429) -> ("States Out"=w428:string)  [unwired: 14 in]
      }
      frame "UI: Format Available" {
        n146 = Unbundle By Name(w446) -> ("refs.available"=w433:refnum<vi>)  [unwired: 1 out]
        n147 = property class="LstBox (strict)"(reference=w433) -> (reference out=w432:refnum<vi>, "Item Names"=w431:string[])  [unwired: 1 in, 1 out]
        n148 = Array Size(array=w431) -> (size(s)=w438:i32)
        n149 = call "Is Value Changed.vim"("value"=w438) -> ("changed or first call?"=w437:bool)
        n150 = In Range and Coerce(upper limit=9, x=w438, lower limit=0) -> (coerced(x)=w441:i32, In Range?=w440:bool)
        n151 = Not(x=w440) -> (.not. x?=w439:bool)
        n152 = property class="LstBox (strict)"(reference=w432, error in=w444, "Item Names"=w431, "Number of Rows"=w441, "Scrollbar Visible"=w439, "Value"=-1) -> (reference out=w435:refnum<vi>, error out=w436:errorcluster)
        n153 = case shown="True" w437 {
          tunnel: w436 -> [w449 w453]
          tunnel: w435 -> [_ w452]
          tunnel: [w449 w450] -> w434
          frame False {
          }
          frame True {
            n154 = property class="LstBox (strict)"(reference=w452, error in=w453, "Top Row"=0) -> (error out=w450:errorcluster)  [unwired: 1 out]
          }
        }
        n155 = call <vilib>:"Add State(s) to Queue__jki_lib_state_machine.vi"("State(s) in (\"\")"=w448) -> ("States Out"=w447:string)  [unwired: 14 in]
      }
      frame "---------- Macro ----------" {
        # "Do not put any code in this frame.\n(It is a separator no-op. You can make a copy of this frame to create a new Macro frame)"
        n156 = call <vilib>:"Add State(s) to Queue__jki_lib_state_machine.vi"("State(s) in (\"\")"=w458) -> ("States Out"=w457:string)  [unwired: 14 in]
      }
      frame "Macro: Initialize" {
        # "Initialization Macro\n(This is called once, when the VI starts)"
        n157 = call <vilib>:"Add State(s) to Queue__jki_lib_state_machine.vi"("State(s) in Front (\"\")"="Data: Initialize\nData: Get Sub-refs\nInitialize Core Data\nEvents: Register\nUI: Initialize\nUI: Selection Change Visible >> false\nUI: List Change Visible >> false\nUI: Set Row Count\nUI: Clear List", "State(s) in (\"\")"=w464) -> ("States Out"=w463:string)  [unwired: 13 in]
      }
      frame "Macro: Exit" {
        # "Exit Macro\n(This is called once, when the VI exits)"
        n158 = Unbundle By Name(w472) -> ("Core.Close Panel on Exit?"=w467:bool)
        n159 = call <vilib>:"Conditional State String__jki_lib_state_machine.vi"("Do State(s)?"=w467, "State"="UI: Front Panel State >> Close") -> ("State Out"=w466:string)  [unwired: 7 in]
        n160 = call <vilib>:"Add State(s) to Queue__jki_lib_state_machine.vi"("State(s) in (\"\")"=w466, "State(s) at Back (\"\")"="UI: Uninitialize\nData: Cleanup\nEvents: Unregister\nExit") -> ("States Out"=w470:string)  [unwired: 13 in]
        n161 = call <vilib>:"Add State(s) to Queue__jki_lib_state_machine.vi"("State(s) in Front (\"\")"=w470, "State(s) in (\"\")"=w474) -> ("States Out"=w473:string)  [unwired: 13 in]
      }
      frame "---------- Actions ----------" {
        # "Template Separator\n(You can make a copy of, or modify, this frame)"
        n162 = call <vilib>:"Add State(s) to Queue__jki_lib_state_machine.vi"("State(s) in (\"\")"=w479) -> ("States Out"=w478:string)  [unwired: 14 in]
      }
      frame "Actions: Add Selection" {
        n163 = Unbundle By Name(w495) -> ("class"=w482:refnum<class "selection_dropdown.lvclass">, "refs.selection"=w486:refnum<vi>, "refs.list"=w494:refnum<vi>)
        n164 = Unbundle By Name(w482) -> ("filter list event"=w481:refnum<user-event>)
        n165 = property class="LstBox (strict)"(reference=w494, error in=w488) -> (reference out=w490:refnum<vi>, error out=w489:errorcluster, "Item Names"=w491:string[])
        n166 = Build Array (concatenate)(w491, w492) -> (w480:string[])
        n167 = property class="LstBox (strict)"(reference=w490, error in=w489, "Item Names"=w480, "Value"=-1) -> (error out=w487:errorcluster)  [unwired: 1 out]
        n168 = property class="Str"(reference=w486, error in=w487, "Value"="") -> (error out=w484:errorcluster)  [unwired: 1 out]
        n169 = Generate User Event(user event=w481, event data cluster=w480, error in=w484) -> (error out=w483:errorcluster)  [unwired: 1 in, 1 out]
        n170 = call <vilib>:"Add State(s) to Queue__jki_lib_state_machine.vi"("State(s) in (\"\")"=w498) -> ("States Out"=w497:string)  [unwired: 14 in]
      }
      frame "Actions: Delete From List" {
        n171 = Unbundle By Name(w511) -> ("class"=w501:refnum<class "selection_dropdown.lvclass">, "refs.list"=w510:refnum<vi>)
        n172 = Unbundle By Name(w501) -> ("filter list event"=w500:refnum<user-event>)
        n173 = property class="LstBox (strict)"(reference=w510, error in=w506) -> (reference out=w508:refnum<vi>, error out=w507:errorcluster, "Item Names"=w505:string[], "Value"=w504:i32)
        n174 = Delete From Array(array=w505, index=w504) -> (array with subset deleted=w499:string[])  [unwired: 1 in, 1 out]
        n175 = property class="LstBox (strict)"(reference=w508, error in=w507, "Item Names"=w499, "Value"=-1) -> (error out=w503:errorcluster)  [unwired: 1 out]
        n176 = Generate User Event(user event=w500, event data cluster=w499, error in=w503) -> (error out=w502:errorcluster)  [unwired: 1 in, 1 out]
        n177 = call <vilib>:"Add State(s) to Queue__jki_lib_state_machine.vi"("State(s) in (\"\")"=w514) -> ("States Out"=w513:string)  [unwired: 14 in]
      }
      frame "Actions: Filter Avail" {
        n178 = Unbundle By Name(w523) -> ("refs.available"=w521:refnum<vi>, "avail set"=w515:string[])
        n179 = To Lower Case(string=w515) -> (all lower case string=w518:string[])
        n180 = To Lower Case(string=w522) -> (all lower case string=w517:string)
        n181 = for {
          tunnel: w518 -> [w530] mode=indexing
          tunnel: w517 -> [w531]
          tunnel: [w527] -> w516 mode=indexing if=w528
          tunnel: w515 -> [w527] mode=indexing
          n182 = Match Pattern(string=w530, regular expression=w531) -> (offset past match=w529:i32)  [unwired: 1 in, 3 out]
          n183 = Greater Or Equal To 0?(x=w529) -> (x >= 0?=w528:bool)
        }
        n184 = property class="LstBox (strict)"(reference=w521, error in=w520, "Item Names"=w516) -> (error out=w519:errorcluster)  [unwired: 1 out]
        n185 = call <vilib>:"Add State(s) to Queue__jki_lib_state_machine.vi"("State(s) in (\"\")"=w526) -> ("States Out"=w525:string)  [unwired: 14 in]
      }
    }
  }
